vi "Thrust_vs_rpm.vi"() -> ()   [LabVIEW 2023]
uses:
  <vilib>/Analysis/NI_AALPro.lvlib
panel:
  out "B/P":dbl
  out "R/G":dbl
  out "Saved as":path caption="Filename Out"
  in  "Save file":bool=TRUE caption="Enable"
  out "Total thrust":dynamicdata(graph)
  out "Best Polynomial Fit":dbl[](array[numeric])
  out "Polynomial Coefficients":dbl[](array[numeric])
  in  "stop":bool
  out "Voltage":dynamicdata(graph)
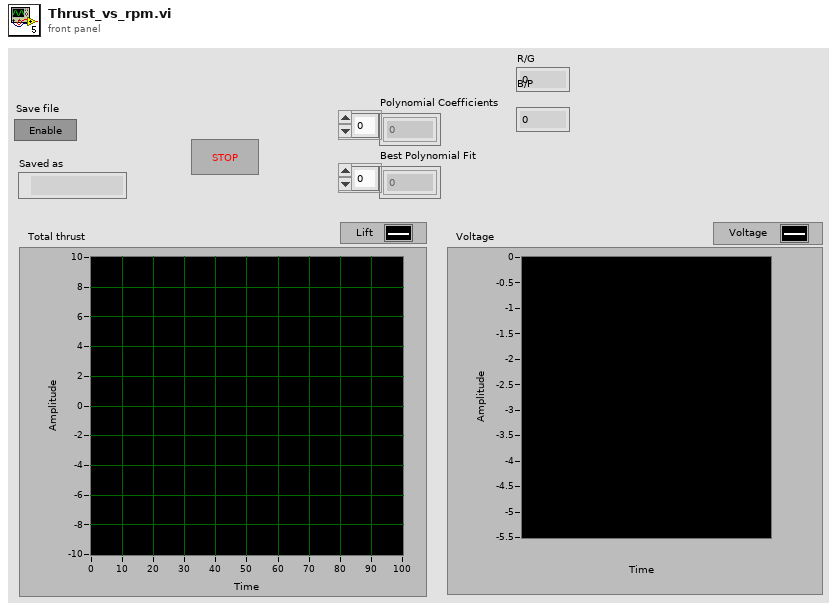
[diagram p1: front panel]
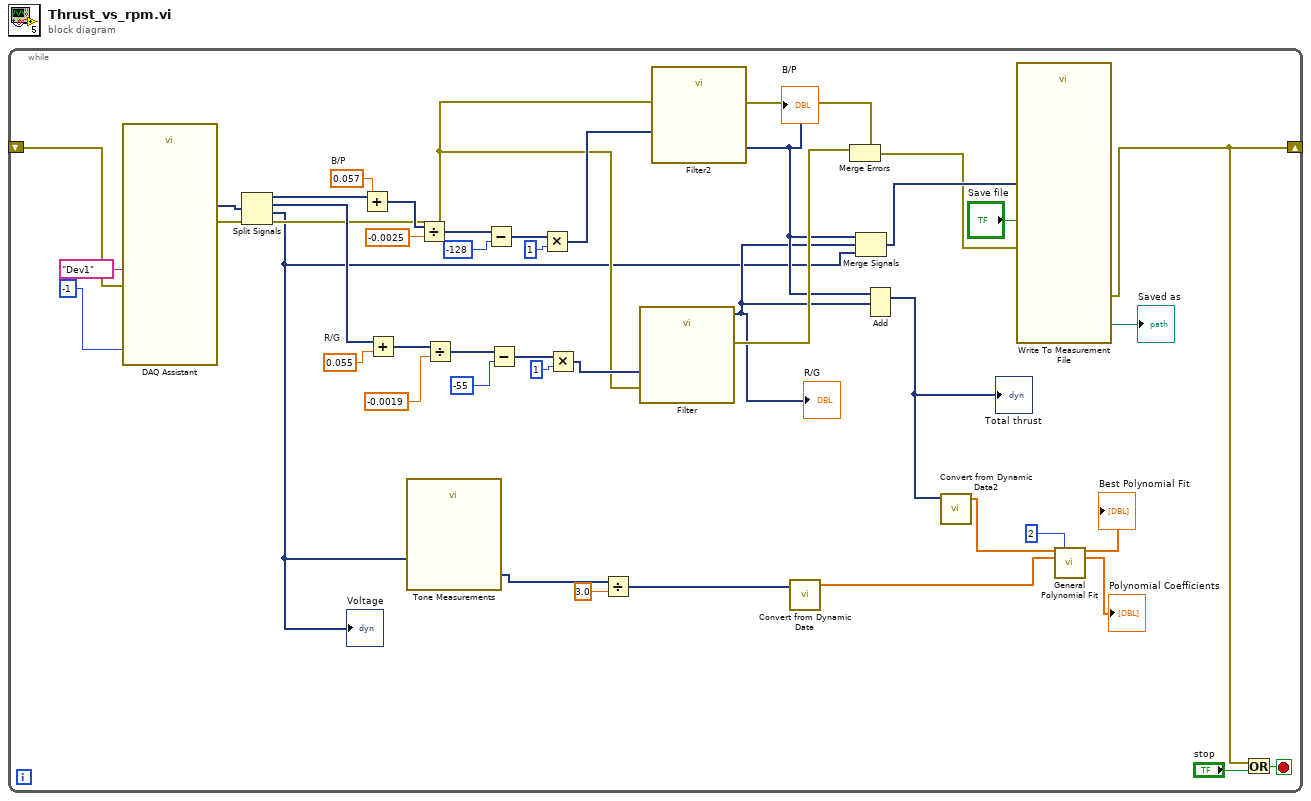
[diagram p0: block diagram]
diagram:
  n1 = while {
    shift-right: [w16] -> _
    shift-left: _ -> [w24]
    stop <- w14 stop-if-true
    w41 = 0.057  # B/P
    w42 = 0.055  # R/G
    n2 = call "DAQ Assistant"("timeout (s)"=-1, "error in"=w24, "device name"=tag "Dev1") -> ("data"=w38:dynamicdata, "error out"=w18:errorcluster)  [unwired: 13 in, 2 out]
    n3 = Split Signals(w38) -> (w36:dynamicdata, w37:dynamicdata, w6:dynamicdata)  [unwired: 4 in, 1 out]
    "Voltage" <- w6
    n4 = Add(x=w36, y=w41) -> (x+y=w44:dynamicdata)
    n5 = Add(x=w37, y=w42) -> (x+y=w43:dynamicdata)
    n6 = call "Tone Measurements"("Signals"=w6) -> ("Frequency"=w5:dynamicdata)  [unwired: 9 in, 1 out]
    n7 = Divide(x=w44, y=-0.0025) -> (x/y=w35:dynamicdata)
    n8 = Divide(x=w43, y=-0.0019) -> (x/y=w33:dynamicdata)
    n9 = Subtract(x=w35, y=-128) -> (x-y=w29:dynamicdata)
    n10 = Subtract(x=w33, y=-55) -> (x-y=w28:dynamicdata)
    n11 = Multiply(x=w29, y=1) -> (x*y=w23:dynamicdata)
    n12 = Multiply(x=w28, y=1) -> (x*y=w27:dynamicdata)
    n13 = Divide(x=w5, y=3.0) -> (x/y=w3:dynamicdata)
    n14 = call "Filter"("error in (no error)"=w18, "Signal"=w27) -> ("error out"=w21:errorcluster, "Filtered Signal"=w10:dynamicdata)  [unwired: 8 in]
    "R/G" <- w10
    n15 = call "Filter2"("error in (no error)"=w18, "Signal"=w23) -> ("error out"=w20:errorcluster, "Filtered Signal"=w17:dynamicdata)  [unwired: 8 in]
    "B/P" <- w17
    n16 = call "Convert from Dynamic Data"("Dynamic Data Type"=w3) -> ("Array"=w2:dbl[])  [unwired: 3 in]
    n17 = Merge Errors(w21, w20) -> (w19:errorcluster)
    n18 = Merge Signals(w17, w10, w6) -> (w25:dynamicdata)
    n19 = Add(1:w10, 2:w17) -> (0:w7:dynamicdata)  [unwired: 1 in, 1 out]
    "Total thrust" <- w7
    n20 = call "Convert from Dynamic Data2"("Dynamic Data Type"=w7) -> ("Array"=w13:dbl[])  [unwired: 3 in]
    n21 = call "Write To Measurement File"("Signals"=w25, "Enable"="Save file", "error in (no error)"=w19) -> ("Filename Out"=→"Saved as":path, "error out"=w16:errorcluster)  [unwired: 14 in, 1 out]
    n22 = call <vilib>:"General Polynomial Fit.vi"("Y"=w13, "polynomial order"=2, "X"=w2) -> ("Best Polynomial Fit"=→"Best Polynomial Fit":dbl[], "Polynomial Coefficients"=→"Polynomial Coefficients":dbl[])  [unwired: 9 in, 2 out]
    n23 = Or(x=w16, y="stop") -> (x .or. y?=w14:bool)
  }
